vi "Clear Bad Data.vi"(11 "Waveform IN":dbl[](array[numeric])) -> (3 "Waveform out":dbl[](array[numeric]))   [LabVIEW 2011]
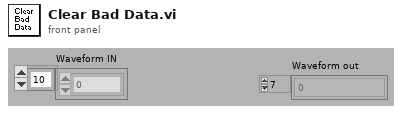
[diagram p1: front panel]
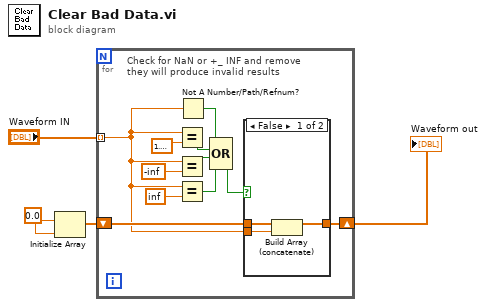
[diagram p0: block diagram]
diagram:
  w3 = 0.0
  n1 = Initialize Array(w3, w3) -> (w4:dbl[])
  n2 = for {
    shift-right: [w11] -> w1
    shift-left: w4 -> [w12]
    tunnel: "Waveform IN" -> [w6] mode=indexing
    # "Check for NaN or +_ INF and remove\nthey will produce invalid results"
    n3 = Equal?(x=w6, y=1.1447298858494002) -> (x = y?=w8:bool)
    n4 = Equal?(x=w6, y=-inf) -> (x = y?=w15:bool)
    n5 = Equal?(x=w6, y=inf) -> (x = y?=w14:bool)
    n6 = Not A Number/Path/Refnum?(number/path/refnum=w6) -> (NaN/Path/Refnum?=w5:bool)
    n7 = Compound Arithmetic op=OR(w5, w8, w15, w14) -> (w13:bool)
    n8 = case shown="False" w13 {
      tunnel: w12 -> [w18 w19]
      tunnel: [w17 w19] -> w11
      tunnel: w6 -> [w16 _]
      frame False {
        n9 = Build Array (concatenate)(w18, w16) -> (w17:dbl[])
      }
      frame True {
      }
    }
  }
  "Waveform out" <- w1
